vi "MS5607_GetCaliByte.vi"(8 "error in (no error)":errorcluster, 11 "Numeric":u8) -> (0 "error out":errorcluster, 3 "Calibration Values":T1)   [LabVIEW 2016]
uses:
  <vilib>/myRIO/Instrument Drivers/Onboard IO/I2C/vis/Configure.vi
  <vilib>/myRIO/Instrument Drivers/Onboard IO/I2C/vis/Write.vi
  <vilib>/myRIO/Instrument Drivers/Onboard IO/I2C/vis/Read.vi
  <vilib>/myRIO/Instrument Drivers/Onboard IO/I2C/vis/Smart Open.vi
  <vilib>/Utility/error.llb/Error Cluster From Error Code.vi
  <vilib>/myRIO/Common/Instrument Driver Framework/myRIO v1.0/I2C/vis/myRIO v1.0 Configure I2C.vi
  <vilib>/myRIO/Common/Instrument Driver Framework/myRIO v1.0/I2C/vis/myRIO v1.0 Write I2C.vi
  <vilib>/myRIO/Common/Instrument Driver Framework/myRIO v1.0/I2C/vis/myRIO v1.0 Read I2C.vi
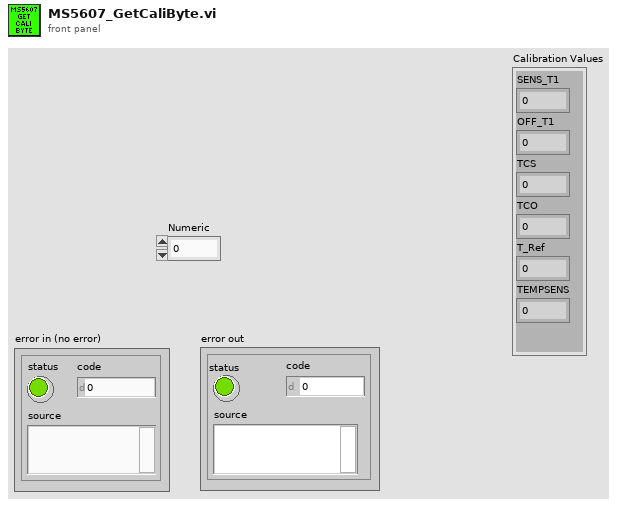
[diagram p1: front panel]
types:
  T1 = cluster{"SENS_T1":u16, "OFF_T1":u16, "TCS":u16, "TCO":u16, "T_Ref":u16, "TEMPSENS":u16}
  T2 = cluster{"[0]":u16, "[1]":u16, "[2]":u16, "[3]":u16, "[4]":u16, "[5]":u16}
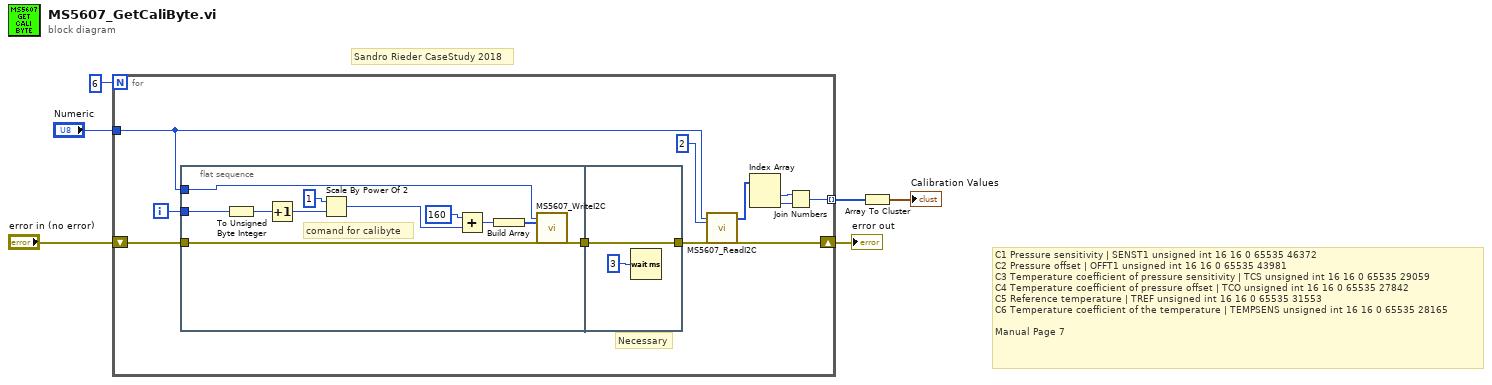
[diagram p0: block diagram]
diagram:
  # "Sandro Rieder CaseStudy 2018"
  # "C1 Pressure sensitivity | SENST1 unsigned int 16 16 0 65535 46372 \nC2 Pressure offset | OFFT1 unsigned int 16 16 0 65535 43981 \nC3 Temperature coefficient of pressure sensitivity | TCS unsigned int 16 16 0 65535 29059 \nC4 Temperature coefficient of pressure offset | TCO unsigned int 16 16 0 65535 27842 \nC5 Reference temperature | TREF unsigned int 16 16 0 65535 31553 \nC6 Temperature coefficient of the temperature | TEMPSENS unsigned int 16 16 0 65535 28165\n\nManual Page 7"
  n1 = for {
    N: 6 -> [_]
    tunnel: "Numeric" -> [w8]
    shift-right: [w10] -> w3
    shift-left: "error in (no error)" -> [w13]
    tunnel: [w16] -> w5 mode=indexing
    i -> [w17]
    # "Necessary"
    n2 = flat-sequence {
      tunnel: w17 -> [w24]
      tunnel: w8 -> [w20]
      tunnel: w13 -> [w19]
      tunnel: [w18] -> w12
      tunnel: [w30] -> w11
      tunnel: w12 -> [w30]
      frame #0 {
        # "comand for calibyte"
        n3 = To Unsigned Byte Integer(number=w24) -> (unsigned 8bit integer=w22:u8)
        n4 = Increment(x=w22) -> (x+1=w23:u8)
        n5 = Scale By Power Of 2(n=i16 1, x=w23) -> (x*2^n=w27:u8)
        n6 = Add(x=u8 160, y=w27) -> (x+y=w26:u8)
        n7 = Build Array(w26) -> (w21:u8[])
        n8 = call "MS5607_WriteI2C.vi"("Slave Address (7-bit)"=w20, "Bytes to Write"=w21, "error in (no error)"=w19) -> ("error out"=w18:errorcluster)  [unwired: 24 in]
      }
      frame #1 {
        n9 = Wait (ms)(milliseconds to wait=u32 3 ("millisecond timer value")) -> ()  [unwired: 1 out]
      }
    }
    n10 = call "MS5607_ReadI2C.vi"("Slave Address (7-bit)"=w8, "Byte Count"=u32 2, "error in (no error)"=w11) -> ("Bytes Read"=w9:u8[], "error out"=w10:errorcluster)  [unwired: 23 in]
    n11 = Index Array(array=w9) -> (element #1=w15:u8, element #2=w14:u8)  [unwired: 2 in]
    n12 = Join Numbers(hi=w15, lo=w14) -> ((hi.lo)=w16:u16)
  }
  "error out" <- w3
  n13 = Array To Cluster(array=w5) -> (cluster=→"Calibration Values":T2)
